vi "Read RT Info.vi"(8 "error in (no error)":errorcluster, 11 "String":string="0.0.0.0") -> (0 "error out":errorcluster, 3 "Target Info":T1)   [LabVIEW 2015]
uses:
  <vilib>/nisyscfg/Close (System).vi
  <vilib>/nisyscfg/nisyscfg.lvlib
  <resource>/objmgr/nisysapi.rc
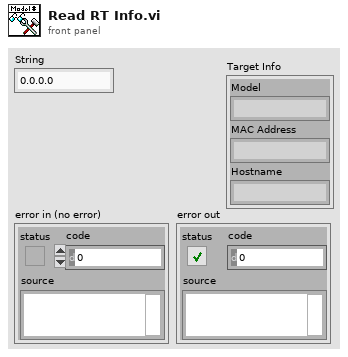
[diagram p1: front panel]
types:
  T1 = cluster{"Model":string, "MAC Address":string, "Hostname":string}
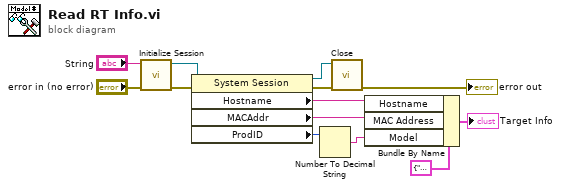
[diagram p0: block diagram]
diagram:
  n1 = call <vilib>:"Initialize Session.vi"("error in (no error)"="error in (no error)", "Target (localhost)"="String") -> ("error out"=w10:errorcluster, "Session out"=w13:refnum<k21>)  [unwired: 8 in]
  n2 = property class="System Session"(reference=w13, error in=w10) -> (reference out=w9:refnum<k21>, error out=w8:errorcluster, "Hostname"=w2:string, "MACAddr"=w5:string, "ProdID"=w4:i32)
  n3 = Number To Decimal String(number=w4) -> (decimal integer string=w3:string)  [unwired: 1 in]
  n4 = call-poly <vilib>:"Close.vi"("error in (no error)"=w8, "Session in"=w9) -> ("error out"=→"error out":errorcluster)  [unwired: 9 in]
  n5 = Bundle By Name(cluster=T1 {"Model"="", "MAC Address"="", "Hostname"=""} ("input cluster"), "Hostname"=w2, "MAC Address"=w5, "Model"=w3) -> (→"Target Info":T1)
